vi "Sweep Keithley 2400.vi"(6 "Ramp Time (s)":dbl=100.0, 9 "Gate Step [V]":dbl=0.01, 10 "final gate voltage (V)":dbl=-1.0 format="%_6f", 11 "KEITHLEY 2400 GPIB Address":string="13") -> (3 "set voltage  (V)":dbl=-1.0 format="%_3f", 8 "GATE Settling \nTime [ms]":dbl=100.0 format="%#_6f")   [LabVIEW 2021]
panel:
  out "Keithley Status (Voltage, Current, etc)":string="-1.000000E+00,-8.804654E-02,+9.910000E+37,+4.142446E+04,+2.150800E+04\n"
  out "Step Wait (ms)":dbl=890.0990099009902
  in  "panic button":bool
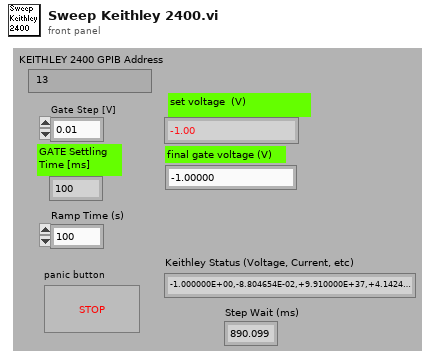
[diagram p1: front panel]
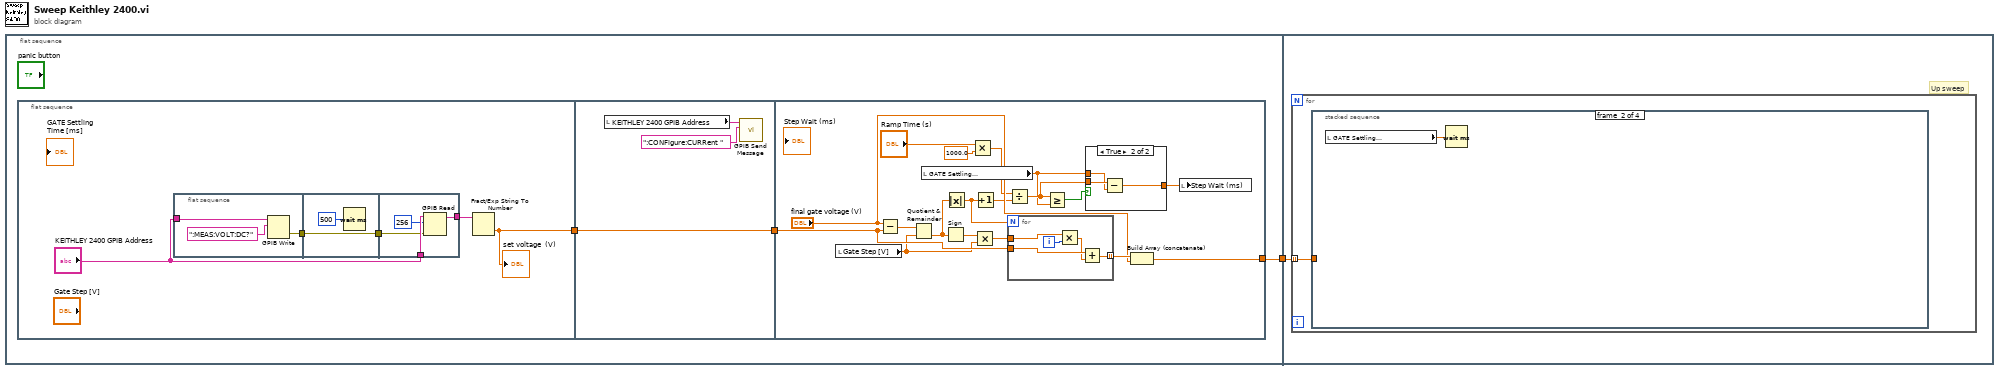
[diagram p0: block diagram]
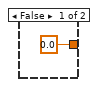
[diagram p2: hidden frame]
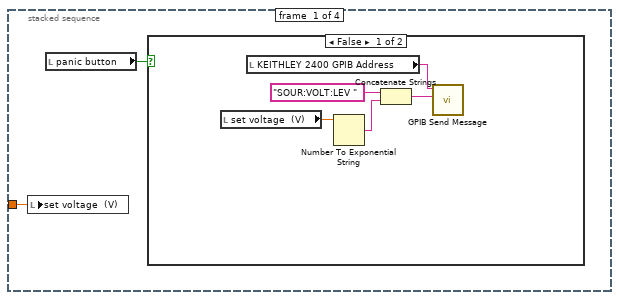
[diagram p3: hidden frame]
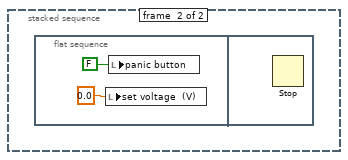
[diagram p5: hidden frame]
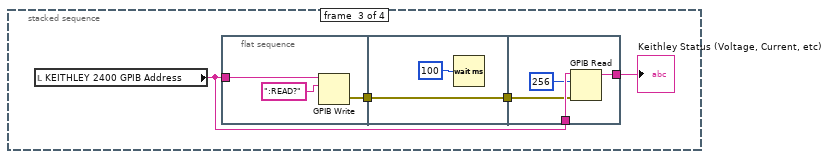
[diagram p6: hidden frame]
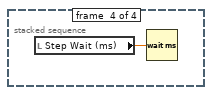
[diagram p7: hidden frame]
diagram:
  n1 = flat-sequence {
    tunnel: [w2] -> w1
    tunnel: w1 -> [w49]
    frame #0 {
      n2 = flat-sequence {
        tunnel: [w5] -> w4
        tunnel: w4 -> [w21]
        tunnel: [w21] -> w3
        tunnel: w3 -> [w34]
        tunnel: [w32] -> w2
        frame #0 {
          n3 = flat-sequence {
            tunnel: "KEITHLEY 2400 GPIB Address" -> [w12]
            tunnel: [w10] -> w9
            tunnel: w9 -> [w13]
            tunnel: [w13] -> w8
            tunnel: "KEITHLEY 2400 GPIB Address" -> [w18]
            tunnel: w8 -> [w16]
            tunnel: [w15] -> w7
            frame #0 {
              n4 = GPIB Write(0:w12, 1:":MEAS:VOLT:DC?" ("data")) -> (6:w10:errorcluster)  [unwired: 3 in, 1 out]
            }
            frame #1 {
              n5 = Wait (ms)(milliseconds to wait=u32 500) -> ()  [unwired: 1 out]
            }
            frame #2 {
              n6 = GPIB Read(0:w18, 1:256 ("byte count"), 3:w16) -> (5:w15:string)  [unwired: 2 in, 2 out]
            }
          }
          n7 = Fract/Exp String To Number(string=w7) -> (number=w5:dbl)  [unwired: 3 in, 1 out]
          "set voltage  (V)" <- w5
        }
        frame #1 {
          n8 = local read "KEITHLEY 2400 GPIB Address"() -> (w20:string)
          n9 = call "GPIB Send Message.vi"("address string"=w20, "write buffer"=":CONFigure:CURRent ") -> ()  [unwired: 5 in, 3 out]
        }
        frame #2 {
          n10 = local read "Gate Step [V]"() -> (w33:dbl)
          n11 = Subtract(x="final gate voltage (V)", y=w34) -> (x-y=w39:dbl)
          n12 = Quotient & Remainder(x=w39, y=w33) -> (floor(x/y)=w37:dbl)  [unwired: 1 out]
          n13 = local read "GATE Settling \nTime [ms]"() -> (w23:dbl)
          n14 = Sign(1:w37) -> (0:w35:dbl)
          n15 = Absolute Value(x=w37) -> (abs(x)=w26:dbl)
          n16 = Multiply(x="Ramp Time (s)", y=1000.0) -> (x*y=w28:dbl)
          n17 = Multiply(x=w35, y=w33) -> (x*y=w36:dbl)
          n18 = Increment(x=w26) -> (x+1=w27:dbl)
          n19 = for {
            N: w26 -> [_]
            tunnel: w34 -> [w48]
            tunnel: [w46] -> w38 mode=indexing
            tunnel: w36 -> [w44]
            i -> [w47]
            n20 = Multiply(x=w44, y=w47) -> (x*y=w45:dbl)
            n21 = Add(x=w48, y=w45) -> (x+y=w46:dbl)
          }
          n22 = Divide(x=w28, y=w27) -> (x/y=w24:dbl)
          n23 = Greater Or Equal?(x=w24, y=w23) -> (x >= y?=w25:bool)
          n24 = case shown="True" w25 {
            tunnel: w24 -> [_ w43]
            tunnel: w23 -> [_ w42]
            tunnel: [0.0 w41] -> w22
            frame False {
            }
            frame True {
              n25 = Subtract(x=w43, y=w42) -> (x-y=w41:dbl)
            }
          }
          n26 = Build Array (concatenate)(w38, "final gate voltage (V)") -> (w32:dbl[])
          n27 = local write "Step Wait (ms)"(w22) -> ()
        }
      }
    }
    frame #1 {
      # "Up sweep"
      n28 = for {
        tunnel: w49 -> [w50] mode=indexing
        n29 = stacked-sequence {
          tunnel: w50 -> [w52 _ _ _]
          frame #0 {
            n30 = local write "set voltage  (V)"(w52) -> ()
            n31 = local read "panic button"() -> (w51:bool)
            n32 = case shown="False" w51 {
              frame False {
                n33 = local read "set voltage  (V)"() -> (w55:dbl)
                n34 = local read "KEITHLEY 2400 GPIB Address"() -> (w54:string)
                n35 = Number To Exponential String(number=w55) -> (E-format string=w56:string)  [unwired: 3 in]
                n36 = Concatenate Strings("SOUR:VOLT:LEV ", w56) -> (w53:string)
                n37 = call "GPIB Send Message.vi"("address string"=w54, "write buffer"=w53) -> ()  [unwired: 5 in, 3 out]
              }
              frame True {
                n38 = stacked-sequence {
                  frame #0 {
                    # "sweep to zero"
                  }
                  frame #1 {
                    n39 = flat-sequence {
                      frame #0 {
                        n40 = local write "set voltage  (V)"(0.0 ("Gate (V)")) -> ()
                        n41 = local write "panic button"(FALSE ("STOP")) -> ()
                      }
                      frame #1 {
                        n42 = Stop() -> ()  [unwired: 1 in]
                      }
                    }
                  }
                }
              }
            }
          }
          frame #1 {
            n43 = local read "GATE Settling \nTime [ms]"() -> (w60:dbl)
            n44 = Wait (ms)(milliseconds to wait=w60) -> ()  [unwired: 1 out]
          }
          frame #2 {
            n45 = local read "KEITHLEY 2400 GPIB Address"() -> (w62:string)
            n46 = flat-sequence {
              tunnel: w62 -> [w67]
              tunnel: [w65] -> w64
              tunnel: w64 -> [w68]
              tunnel: [w68] -> w63
              tunnel: w62 -> [w73]
              tunnel: w63 -> [w71]
              tunnel: [w70] -> w61
              frame #0 {
                n47 = GPIB Write(0:w67, 1:":READ?" ("data")) -> (6:w65:errorcluster)  [unwired: 3 in, 1 out]
              }
              frame #1 {
                n48 = Wait (ms)(milliseconds to wait=u32 100) -> ()  [unwired: 1 out]
              }
              frame #2 {
                n49 = GPIB Read(0:w73, 1:256 ("byte count"), 3:w71) -> (5:w70:string)  [unwired: 2 in, 2 out]
              }
            }
            "Keithley Status (Voltage, Current, etc)" <- w61
          }
          frame #3 {
            n50 = local read "Step Wait (ms)"() -> (w74:dbl)
            n51 = Wait (ms)(milliseconds to wait=w74) -> ()  [unwired: 1 out]
          }
        }
      }
    }
  }
